vi "窗口自动调整.vi-.vi"(4 "error in (no error)":errorcluster, 5 "max？":bool, 6 "border spacing (2 px)":i32=2, 7 "VI Ref (calling VI)":refnum<vi>) -> (0 "error out":errorcluster, 3 "dup VI Ref":refnum<vi>)   [LabVIEW 2020]
doc: "This utility will fit (resize and center) a VI (defined by the \"VI Ref\" input) about the largest decoration in that VI. It will add a border defined by border spacing in units of pixels. If there are no decorations found in the VI it is a no-op and will not produce an error. Unfortunately, this VI can not find locked decorations (yet)."
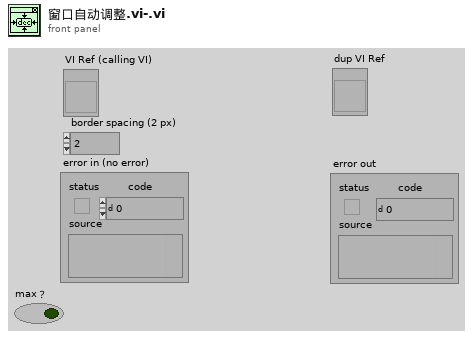
[diagram p1: front panel]
types:
  T1 = typedef "LVRectTypeDef.ctl" = cluster{"Left":i16, "Top":i16, "Right":i16, "Bottom":i16}
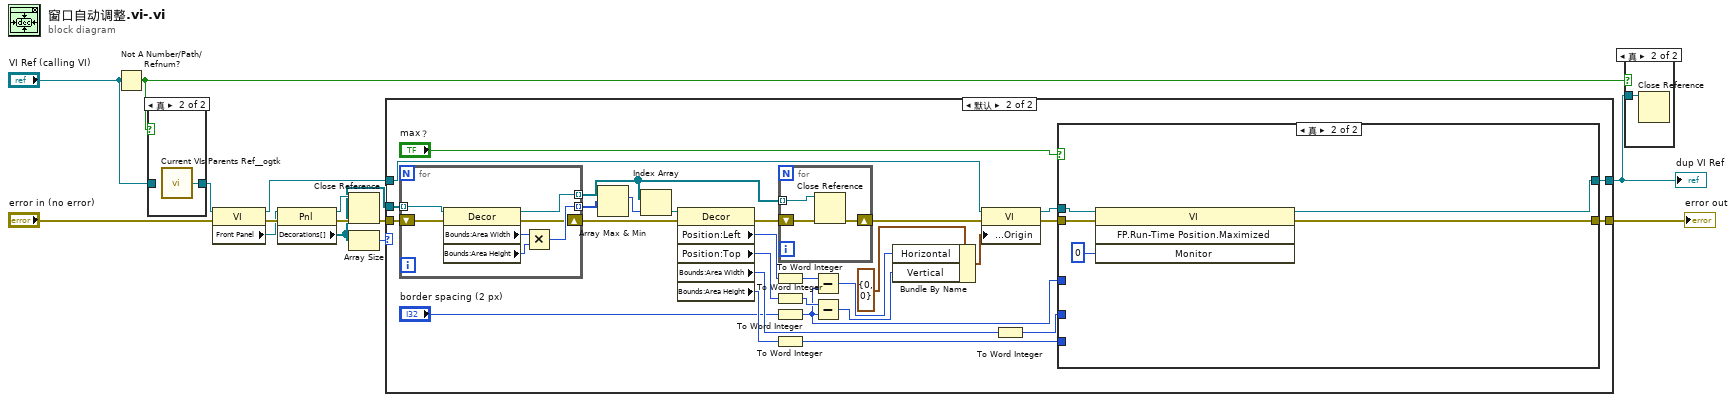
[diagram p0: block diagram]
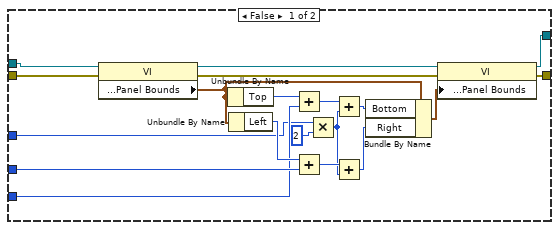
[diagram p5: hidden frame]
diagram:
  n1 = Not A Number/Path/Refnum?(number/path/refnum="VI Ref (calling VI)") -> (NaN/Path/Refnum?=w2:bool)
  n2 = case shown="真" w2 {
    tunnel: [w15 w16] -> w3
    tunnel: "VI Ref (calling VI)" -> [w15 _]
    frame False {
    }
    frame True {
      n3 = call <userlib>:"Current VIs Parents Ref__ogtk.vi"() -> ("Calling VI's Reference"=w16:refnum<vi>)  [unwired: 2 in]
    }
  }
  n4 = property on="Property Node" class="VI"(reference=w3, error in="error in (no error)") -> (reference out=w14:refnum<vi>, error out=w12:errorcluster, "Front Panel"=w9:refnum<vi>)
  n5 = property on="Property Node" class="Pnl"(reference=w9, error in=w12) -> (reference out=w13:refnum<vi>, error out=w11:errorcluster, "Decorations[]"=w6:refnum<vi>[])
  n6 = Close Reference(reference=w13, error in (no error)=w11) -> (error out=w8:errorcluster)
  n7 = Array Size(array=w6) -> (size(s)=w5:i32)
  n8 = case shown="默认" w5 {
    tunnel: w14 -> [w18 w46]
    tunnel: w8 -> [w17 w37]
    tunnel: [w17 w20] -> w7
    tunnel: [w18 w21] -> w1
    tunnel: w6 -> [_ w27]
    frame 0 {
    }
    frame Default {
      n9 = for {
        tunnel: w27 -> [w78] mode=indexing
        tunnel: [w75] -> w36 mode=indexing
        shift-right: [w73] -> w32
        shift-left: w37 -> [w74]
        tunnel: [w72] -> w34 mode=indexing
        n10 = property class="Decor"(reference=w78, error in=w74) -> (reference out=w72:refnum<vi>, error out=w73:errorcluster, "Bounds:Area Width"=w77:u32, "Bounds:Area Height"=w76:u32)
        n11 = Multiply(x=w77, y=w76) -> (x*y=w75:u32)
      }
      n12 = Array Max & Min(array=w36) -> (max index (indices)=w35:i32)  [unwired: 3 out]
      n13 = Index Array(array=w34, index=w35) -> (element=w33:refnum<vi>)
      n14 = property class="Decor"(reference=w33, error in=w32) -> (error out=w31:errorcluster, "Position:Left"=w40:i32, "Position:Top"=w43:i32, "Bounds:Area Width"=w45:u32, "Bounds:Area Height"=w44:u32)  [unwired: 1 out]
      n15 = To Word Integer(number=w40) -> (16bit integer=w24:i16)
      n16 = To Word Integer(number=w43) -> (16bit integer=w23:i16)
      n17 = To Word Integer(number="border spacing (2 px)") -> (16bit integer=w22:i16)
      n18 = To Word Integer(number=w44) -> (16bit integer=w25:i16)
      n19 = for {
        tunnel: w34 -> [w81] mode=indexing
        shift-right: [w79] -> w29
        shift-left: w31 -> [w80]
        n20 = Close Reference(reference=w81, error in (no error)=w80) -> (error out=w79:errorcluster)
      }
      n21 = Subtract(x=w24, y=w22) -> (x-y=w41:i16)
      n22 = Subtract(x=w23, y=w22) -> (x-y=w42:i16)
      n23 = Bundle By Name(cluster=cluster{"Horizontal":i16, "Vertical":i16} {"Horizontal"=0, "Vertical"=0} ("Front Panel Window:Origin"), "Horizontal"=w41, "Vertical"=w42) -> (w38:cluster{"Horizontal":i16, "Vertical":i16})
      n24 = property on="Property Node" class="VI"(reference=w46, error in=w29, "Front Panel Window:Origin"=w38) -> (reference out=w47:refnum<vi>, error out=w28:errorcluster)
      n25 = To Word Integer(number=w45) -> (16bit integer=w26:i16)
      n26 = case shown="真" "max？" {
        tunnel: w47 -> [w65 w70]
        tunnel: w28 -> [w55 w69]
        tunnel: w26 -> [w52 _]
        tunnel: w25 -> [w51 _]
        tunnel: w22 -> [w50 _]
        tunnel: [w49 w68] -> w21
        tunnel: [w48 w67] -> w20
        frame False {
          n27 = property on="Property Node" class="VI"(reference=w65, error in=w55) -> (reference out=w66:refnum<vi>, error out=w54:errorcluster, "Front Panel Window:Panel Bounds"=w57:T1)
          n28 = Unbundle By Name(w57) -> ("Top"=w58:i16)
          n29 = Unbundle By Name(w57) -> ("Left"=w59:i16)
          n30 = Add(x=w58, y=w51) -> (x+y=w63:i16)
          n31 = Add(x=w59, y=w52) -> (x+y=w61:i16)
          n32 = Multiply(x=w50, y=i16 2) -> (x*y=w53:i16)
          n33 = Add(x=w63, y=w53) -> (x+y=w64:i16)
          n34 = Add(x=w61, y=w53) -> (x+y=w62:i16)
          n35 = Bundle By Name(cluster=w57, "Bottom"=w64, "Right"=w62) -> (w60:T1)
          n36 = property on="Property Node" class="VI"(reference=w66, error in=w54, "Front Panel Window:Panel Bounds"=w60) -> (reference out=w49:refnum<vi>, error out=w48:errorcluster)
        }
        frame True {
          n37 = invoke class="VI" method="FP.Run-Time Position.Maximized"(reference=w70, error in=w69, "Monitor"=i16 0 ("显示器")) -> (reference out=w68:refnum<vi>, error out=w67:errorcluster)  [unwired: 1 in, 2 out]
        }
      }
    }
  }
  "error out" <- w7
  "dup VI Ref" <- w1
  n38 = case shown="真" w2 {
    tunnel: w1 -> [_ w82]
    frame False {
    }
    frame True {
      n39 = Close Reference(reference=w82) -> ()  [unwired: 1 in, 1 out]
    }
  }
